vi "exitMaintenance.vi"(8 "error in (no error)":errorcluster, 9 "Parameters":T1, 10 "Model in":refnum<class "Model.lvclass">, 11 "ParkedMaintenanceState in":refnum<class "ParkedMaintenanceState.lvclass">) -> (0 "error out":errorcluster, 2 "Model out":refnum<class "Model.lvclass">, 3 "ParkedMaintenanceState out":refnum<class "ParkedMaintenanceState.lvclass">)   [LabVIEW 2016, in "ParkedMaintenanceState.lvclass"]
uses:
  ParkedMaintenanceState.lvclass
  DataTypes/Topics/CommandExitMaintenance.ctl
  DataTypes/Topics/Parts/CommandId.ctl
  Model/Model.lvclass
  DataTypes/Topics/Parts/DetailedStates.ctl
  DataTypes/Topics/M1M3SupportTopics.lvlib
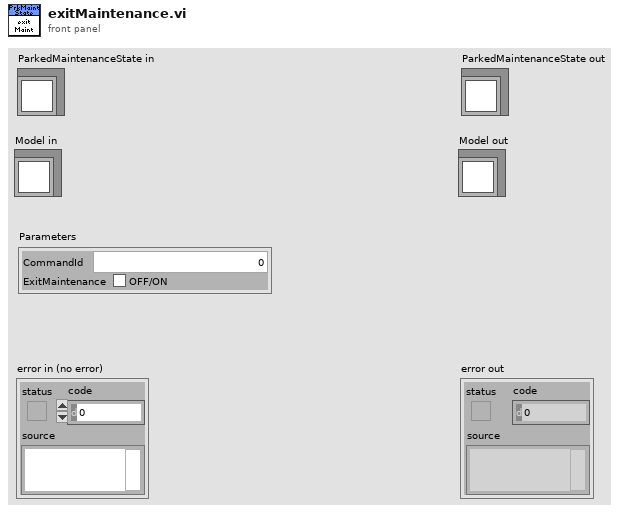
[diagram p1: front panel]
types:
  T1 = typedef "M1M3SupportTopics.lvlib/CommandExitMaintenance.ctl" = cluster{"CommandId":T2, "ExitMaintenance":bool}
  T2 = typedef "M1M3SupportTopics.lvlib/CommandId.ctl" = i32
  T3 = typedef "M1M3SupportTopics.lvlib/DetailedStates.ctl" = enum16{"OfflineState", "InitialState", "StandbyState", "DisabledState", "ParkedState", "FaultState", "ParkedMaintenanceState", "ActiveMaintenanceState"}
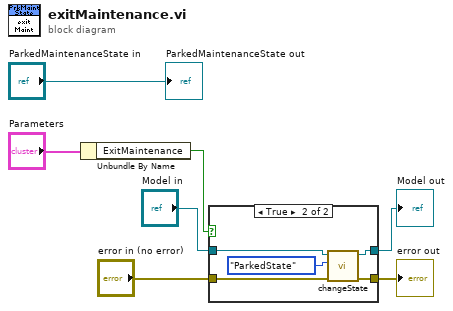
[diagram p0: block diagram]
diagram:
  n1 = Unbundle By Name("Parameters") -> ("ExitMaintenance"=w1:bool)
  n2 = case shown="True" w1 {
    tunnel: "Model in" -> [w9 w14]
    tunnel: [w9 w12] -> w5
    tunnel: "error in (no error)" -> [w8 w11]
    tunnel: [w8 w10] -> w3
    frame False {
    }
    frame True {
      n3 = call "changeState.vi"("error in (no error)"=w11, "DetailedStates"=DetailedStates."ParkedState", "Model in"=w14) -> ("error out"=w10:errorcluster, "Model out"=w12:refnum<class "Model.lvclass">)  [unwired: 7 in]
    }
  }
  "error out" <- w3
  "Model out" <- w5
  "ParkedMaintenanceState out" <- "ParkedMaintenanceState in"
